vi "Depth Frame Read.vi"(8 "error in (no error)":errorcluster, 11 "ROIed Video Frame in":refnum<class "ROIed Video Frame.lvclass">) -> (0 "error out":errorcluster, 2 "Depth Values":dbl[](array[numeric]), 3 "ROIed Video Frame out":refnum<class "ROIed Video Frame.lvclass">, 4 "Average Depth":dbl, 6 "Standard Deviation":dbl)   [LabVIEW 2018, in "ROIed Video Frame.lvclass"]
uses:
  ROIed Video Frame.lvclass
  C:/Users/aaron.jencks/Documents/GitHub/emerson_seed_object_detection/LabVIEW/Projects/Paul's Video Viewer/Classes/Video Frame/Video Frame.lvclass
  33a65961-67c5-4527-ae99-978ca56d9254.vi
  e44e4fe8-f30f-4b2a-9cd0-8f514ca4bcba.vi
  e44e4fe8-f30f-4b2a-9cd0-8f514ca4bcba.vi/d243726d-1b4d-4e39-b745-b4c3b038740c.vi
  Video Frame/Video Frame.lvclass
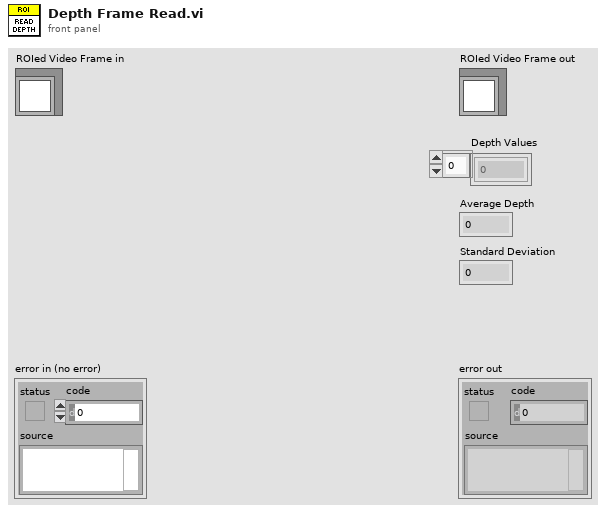
[diagram p1: front panel]
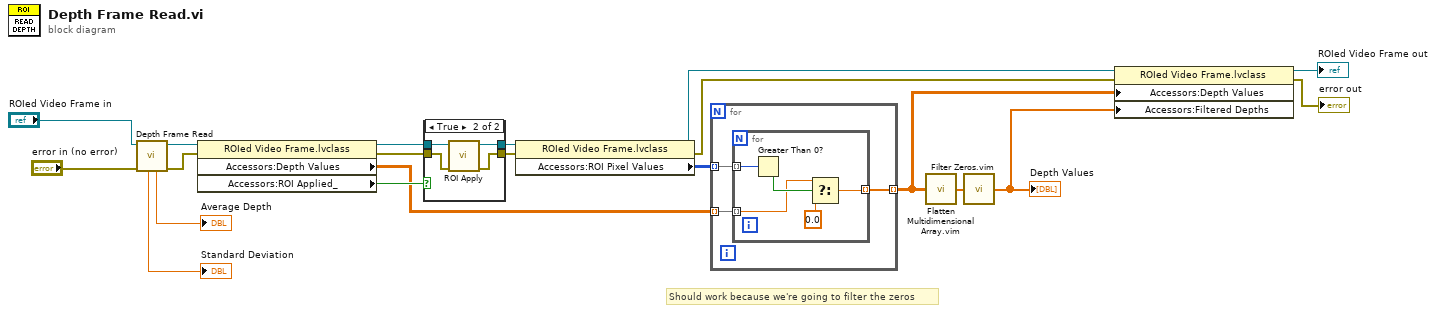
[diagram p0: block diagram]
diagram:
  # "Should work because we're going to filter the zeros"
  n1 = call-parent "Depth Frame Read.vi"("error in (no error)"="error in (no error)", "Video Frame in"="ROIed Video Frame in") -> ("error out"=w15:errorcluster, "Video Frame out"=w18:refnum<class "ROIed Video Frame.lvclass">, "Average Depth"=→"Average Depth":dbl, "Standard Deviation"=→"Standard Deviation":dbl)  [unwired: 5 in, 1 out]
  n2 = property class="ROIed Video Frame.lvclass"(reference=w18, error in=w15) -> (reference out=w16:refnum<class "ROIed Video Frame.lvclass">, error out=w14:errorcluster, "Accessors:Depth Values"=w10:dbl[][], "Accessors:ROI Applied_"=w17:bool)
  n3 = case shown="True" w17 {
    tunnel: w16 -> [w22 w26]
    tunnel: w14 -> [w21 w25]
    tunnel: [w22 w24] -> w13
    tunnel: [w21 w23] -> w12
    frame False {
    }
    frame True {
      n4 = call-dynamic "ROI Apply.vi"("error in (no error)"=w25, "ROIed Video Frame in"=w26) -> ("error out"=w23:errorcluster, "ROIed Video Frame out"=w24:refnum<class "ROIed Video Frame.lvclass">)  [unwired: 8 in]
    }
  }
  n5 = property class="ROIed Video Frame.lvclass"(reference=w13, error in=w12) -> (reference out=w9:refnum<class "ROIed Video Frame.lvclass">, error out=w4:errorcluster, "Accessors:ROI Pixel Values"=w11:u8[][])
  n6 = for {
    tunnel: w11 -> [w29] mode=indexing
    tunnel: w10 -> [w28] mode=indexing
    tunnel: [w27] -> w6 mode=indexing
    n7 = for {
      tunnel: w29 -> [w34] mode=indexing
      tunnel: w28 -> [w32] mode=indexing
      tunnel: [w30] -> w27 mode=indexing
      n8 = Greater Than 0?(x=w34) -> (x > 0?=w33:bool)
      n9 = Select(t=w32, s=w33, f=0.0) -> (s? t:f=w30:dbl)
    }
  }
  n10 = call "Flatten Multidimensional Array.vim"("Array"=w6) -> ("output array"=w7:dbl[])  [unwired: 14 in]
  n11 = call "Filter Zeros.vim"("Array"=w7) -> ("Array Out"=w5:dbl[])  [unwired: 14 in]
  "Depth Values" <- w5
  n12 = property class="ROIed Video Frame.lvclass"(reference=w9, error in=w4, "Accessors:Depth Values"=w6, "Accessors:Filtered Depths"=w5) -> (reference out=→"ROIed Video Frame out":refnum<class "ROIed Video Frame.lvclass">, error out=→"error out":errorcluster)
